vi "Get Temp Dir.vi"(8 "error in":errorcluster, 11 "Control in":refnum<class "Control.lvclass">) -> (0 "error out":errorcluster, 2 "temp directory":path, 3 "Control out":refnum<class "Control.lvclass">)   [LabVIEW 2013, in "Control.lvclass"]
doc: "Get the temporary directory path"
uses:
  Control.lvclass
  <userlib>/_OpenG.lib/file/file.llb/Strip Path - Traditional__ogtk.vi
  <userlib>/_OpenG.lib/file/file.llb/Build Path - Traditional - path__ogtk.vi
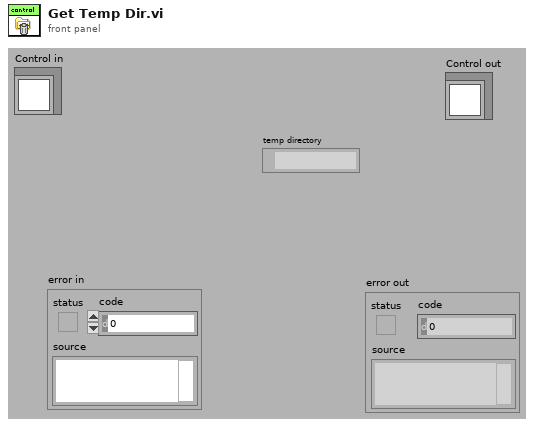
[diagram p1: front panel]
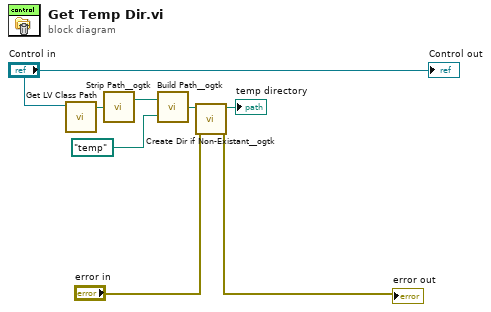
[diagram p0: block diagram]
diagram:
  n1 = call <vilib>:"Get LV Class Path.vi"("object"="Control in") -> ("class path"=w8:path)  [unwired: 1 in, 9 out]
  n2 = call-poly <userlib>:"Strip Path__ogtk.vi"("path"=w8) -> ("stripped path"=w6:path)  [unwired: 1 out]
  n3 = call-poly <userlib>:"Build Path__ogtk.vi"("name or relative path"=path "temp" ("Relative path (.)"), "base path"=w6) -> ("appended path"=w5:path)
  n4 = call <userlib>:"Create Dir if Non-Existant__ogtk.vi"("error in (no error)"="error in", "Directory Path"=w5) -> ("error out"=→"error out":errorcluster, "dup Directory Path"=→"temp directory":path)  [unwired: 1 in, 7 out]
  "Control out" <- "Control in"
